vi "Write Build spec id.vi"(8 "Build spec name":string, 9 "Buid spec section":string, 10 "Target":string, 11 "ProjectItem in":refnum<class "ProjectItem.lvclass">) -> (3 "ProjectItem out":refnum<class "ProjectItem.lvclass">)   [LabVIEW 2019, in "SolutionBuilder.lvlib" / "ProjectItem.lvclass"]
uses:
  ProjectItem.lvclass
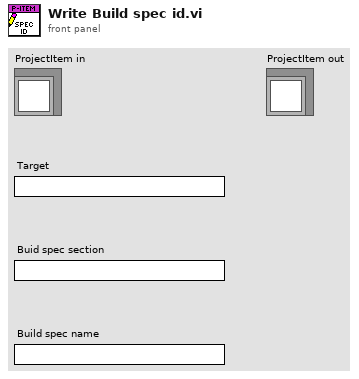
[diagram p1: front panel]
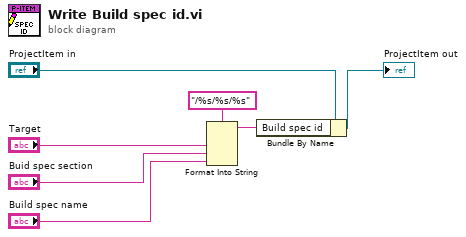
[diagram p0: block diagram]
diagram:
  n1 = Format Into String(format string="/%s/%s/%s", "Target", "Buid spec section", "Build spec name") -> (resulting string=w3:string)  [unwired: 2 in, 1 out]
  n2 = Bundle By Name(cluster="ProjectItem in", "Build spec id"=w3) -> (→"ProjectItem out":refnum<class "ProjectItem.lvclass">)
